vi "Timeout Check.vi"(6 "Start":bool, 8 "error in (no error)":errorcluster, 11 "Detector Manager in":refnum<class "Detector Manager.lvclass">) -> (0 "error out":errorcluster, 2 "Timeout":bool, 3 "Detector Manager out":refnum<class "Detector Manager.lvclass">)   [LabVIEW 2026, in "TALOS.lvlib" / "Detector Manager.lvlib" / "Detector Manager.lvclass"]
uses:
  Detector Manager.lvclass
  Detector Manager.lvclass/Detector Manager.ctl
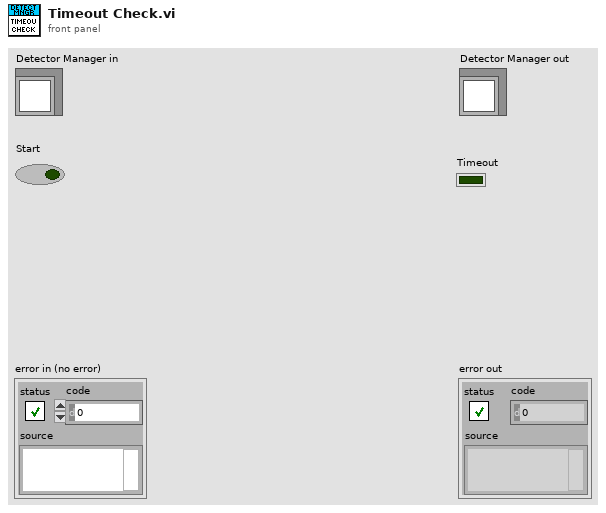
[diagram p1: front panel]
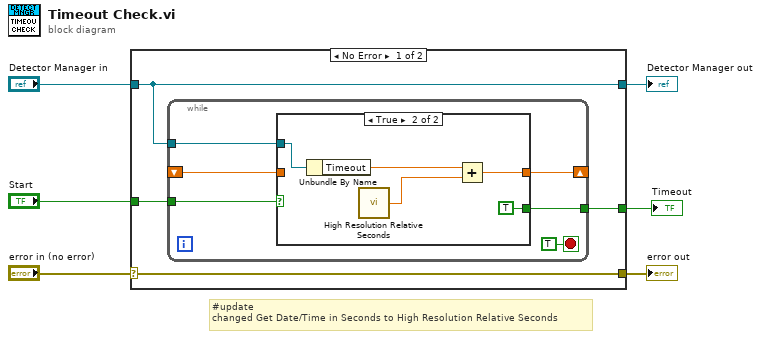
[diagram p0: block diagram]
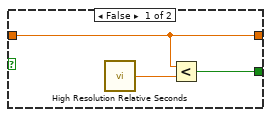
[diagram p2: hidden frame]
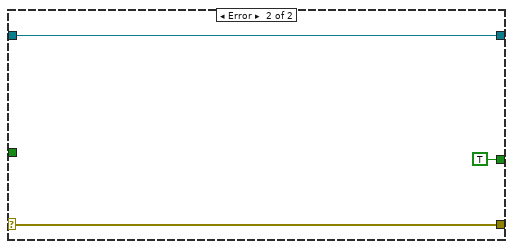
[diagram p3: hidden frame]
diagram:
  # "#update\nchanged Get Date/Time in Seconds to High Resolution Relative Seconds"
  n1 = case shown="No Error" "error in (no error)" {
    selector: "error in (no error)" -> [w10 w27]
    tunnel: [w10 w27] -> w5
    tunnel: [w9 w26] -> w3
    tunnel: "Detector Manager in" -> [w9 w26]
    tunnel: "Start" -> [w8 _]
    tunnel: [w7 TRUE] -> w1
    frame No Error {
      n2 = while {
        tunnel: w9 -> [w15]
        tunnel: w8 -> [w14]
        shift-right: [w13] -> _
        shift-left: _ -> [w12]
        tunnel: [w11] -> w7
        stop <- TRUE stop-if-true
        n3 = case shown="True" w14 {
          tunnel: w15 -> [_ w24]
          tunnel: [w19 w22] -> w13
          tunnel: w12 -> [w19 _]
          tunnel: [w17 TRUE] -> w11
          frame False {
            n4 = call <vilib>:"High Resolution Relative Seconds.vi"() -> ("relative seconds"=w18:dbl)
            n5 = Less?(x=w19, y=w18) -> (x < y?=w17:bool)
          }
          frame True {
            n6 = Unbundle By Name(w24) -> ("Timeout"=w23:dbl)
            n7 = call <vilib>:"High Resolution Relative Seconds.vi"() -> ("relative seconds"=w21:dbl)
            n8 = Add(x=w23, y=w21) -> (x+y=w22:dbl)
          }
        }
      }
    }
    frame Error {
    }
  }
  "error out" <- w5
  "Detector Manager out" <- w3
  "Timeout" <- w1
